vi "SetTemp.vi"(8 "error in (no error)":errorcluster, 10 "Set temp":string="320", 11 "path to XML document":path=path "C:/Users/user/AppData/Roaming/CryoConnector/811187/status.xml") -> (0 "error out":errorcluster)   [LabVIEW 2016]
uses:
  <vilib>/xml/Load XML File.vi
  <vilib>/xml/Close Reference(Node).vi
  <vilib>/xml/NI_XML.lvlib
  <resource>/objmgr/DOMUserDefRef.rc
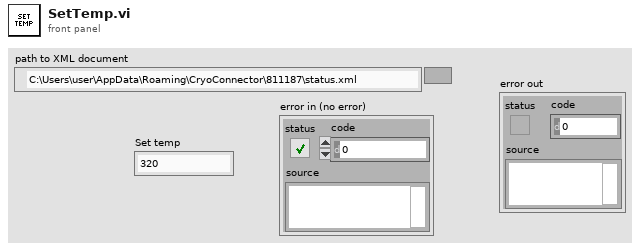
[diagram p1: front panel]
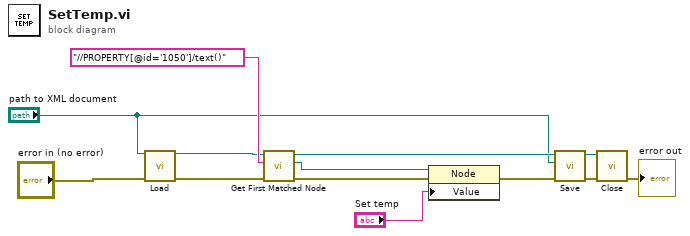
[diagram p0: block diagram]
diagram:
  n1 = call-poly <vilib>:"Load.vi"("path to XML document"="path to XML document", "error in (no error)"="error in (no error)") -> ("DOM document out"=w6:refnum<k20>, "error out"=w11:errorcluster)  [unwired: 11 in, 1 out]
  n2 = call <vilib>:"Get First Matched Node.vi"("error in (no error)"=w11, "XPath expression"="//PROPERTY[@id='1050']/text()", "node in"=w6) -> ("error out"=w2:errorcluster, "node result"=w3:refnum<k20>, "node out"=w10:refnum<k20>)  [unwired: 6 in]
  n3 = property class="Node"(reference=w3, error in=w2, "Value"="Set temp") -> (error out=w1:errorcluster)  [unwired: 1 out]
  n4 = call <vilib>:"Save.vi"("error in (no error)"=w1, "XML file path"="path to XML document", "DOM document in"=w10) -> ("error out"=w8:errorcluster, "DOM document out"=w9:refnum<k20>)  [unwired: 6 in, 1 out]
  n5 = call-poly <vilib>:"Close.vi"("error in (no error)"=w8, "node"=w9) -> ("error out"=→"error out":errorcluster)  [unwired: 7 in]
